vi "Generator_b.vi"(0 "Stop":bool caption="Start/Stop") -> (4 "Generated_Data":dbl caption="Generated Data")   [LabVIEW 2023]
doc: "This VI continuously generate Data and push it to the Acquisition VI.\nTransfer of thet data happens under Simple LV2."
uses:
  Type_Def/Operation_Simple_LV2.ctl
  <vilib>/numeric/Random Number (Range) DBL.vi
panel:
  out "Error_Out":errorcluster
  in  "Error_In":errorcluster
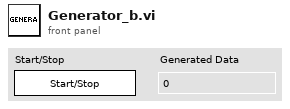
[diagram p1: front panel]
types:
  T1 = typedef "Operation_Simple_LV2.ctl" = u16
  T2 = enum16{"Left Button", "Center Button", "Right Button", "Window Close"}
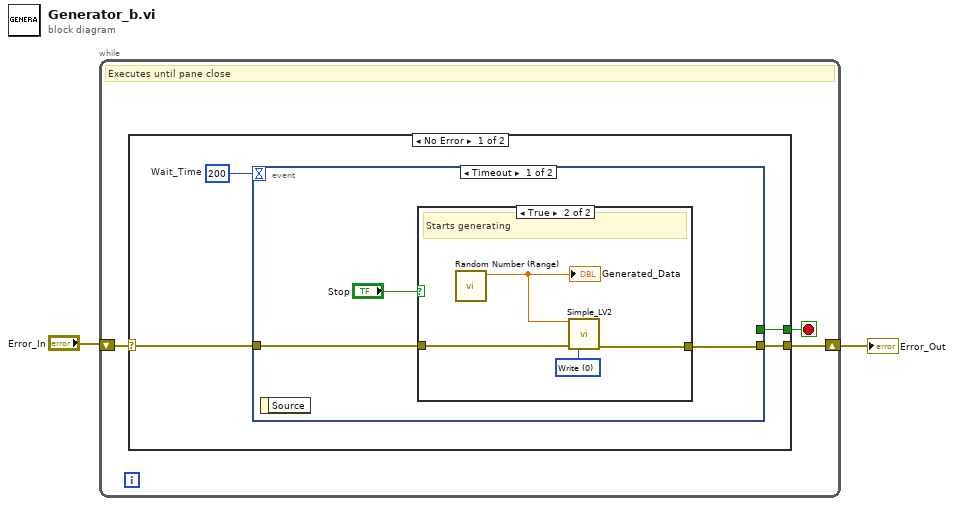
[diagram p0: block diagram]
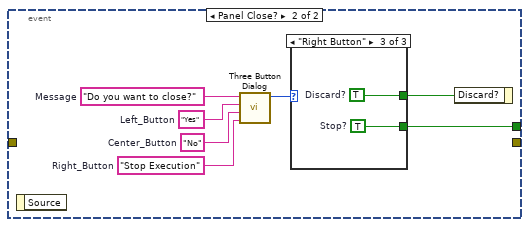
[diagram p3: hidden frame]
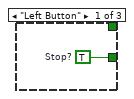
[diagram p4: hidden frame]
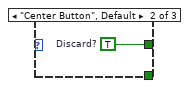
[diagram p5: hidden frame]
diagram:
  n1 = while {
    shift-right: [w3] -> w1
    shift-left: "Error_In" -> [w4]
    stop <- w5 stop-if-true
    # "Executes until pane close"
    n2 = case shown="No Error" w4 {
      selector: w4 -> [w7 w29]
      tunnel: [w8 _] -> w5
      tunnel: [w6 w29] -> w3
      frame No Error {
        w9 = 200  # Wait_Time
        n3 = event shown="[0] Timeout" {
          selector: _ -> [_ _]
          dyn-events: _ -> [_ _]
          timeout: w9 -> [_ _]
          tunnel: [_ w18] -> w8
          tunnel: w7 -> [w12 _]
          tunnel: [w11 _] -> w6
          event Timeout {
            n4 = event-data() -> ()  [unwired: 1 in, 1 out]
            n5 = case shown="True" "Stop" {
              tunnel: w12 -> [w13 w15]
              tunnel: [w13 w14] -> w11
              frame False {
                # "Stop generating"
              }
              frame True {
                w16 = T1 0 items=["Write", "Read"] ("Ring")
                # "Starts generating"
                n6 = call-poly <vilib>:"Random Number (Range).vi"() -> ("number"=w17:dbl)  [unwired: 11 in]
                "Generated_Data" <- w17
                n7 = call "Simple_LV2.vi"("Data_In"=w17, "Error_In"=w15, "Ring"=w16) -> ("Error_Out"=w14:errorcluster)  [unwired: 11 in, 1 out]
              }
            }
          }
          event Panel Close? {
            w21 = "Stop Execution"  # Right_Button
            w22 = "No"  # Center_Button
            w23 = "Yes"  # Left_Button
            w24 = "Do you want to close?"  # Message
            n8 = event-data() -> ()  [unwired: 1 in, 1 out]
            n9 = call <vilib>:"Three Button Dialog.vi"("Right Button Text (\"Cancel\")"=w21, "Center Button Text (\"No\")"=w22, "Left Button Text (\"Yes\")"=w23, "message"=w24) -> ("Which Button?"=w20:T2)  [unwired: 7 in]
            n10 = case shown="\"Right Button\"" w20 {
              tunnel: [_ w26 w27] -> w19
              tunnel: [w25 _ w28] -> w18
              frame "Left Button" {
                w25 = TRUE  # Stop?
              }
              frame "Center Button", Default {
                w26 = TRUE  # Discard?
              }
              frame "Right Button" {
                w27 = TRUE  # Discard?
                w28 = TRUE  # Stop?
              }
            }
            n11 = event-data("Discard?"=w19) -> ()  [unwired: 1 in, 1 out]
          }
        }
      }
      frame Error {
      }
    }
  }
  "Error_Out" <- w1
